vi "VCI Transmit.vi"(6 "Len":u32, 7 "pSend":T1, 8 "error in (no error)":errorcluster, 9 "CANIndex":u32, 10 "DevIndex":u32, 11 "DevType":u32) -> (0 "error out":errorcluster, 3 "function return":u32)   [LabVIEW 2012, in "ControlCAN.lvlib"]
doc: "unsigned int WINAPI VCI_Transmit(unsigned int DevType,unsigned int DevIndex,unsigned int CANIndex,PVCI_CAN_OBJ pSend,unsigned int Len);"
uses:
  ControlCAN.lvlib
  Ginkgo_Driver.dll
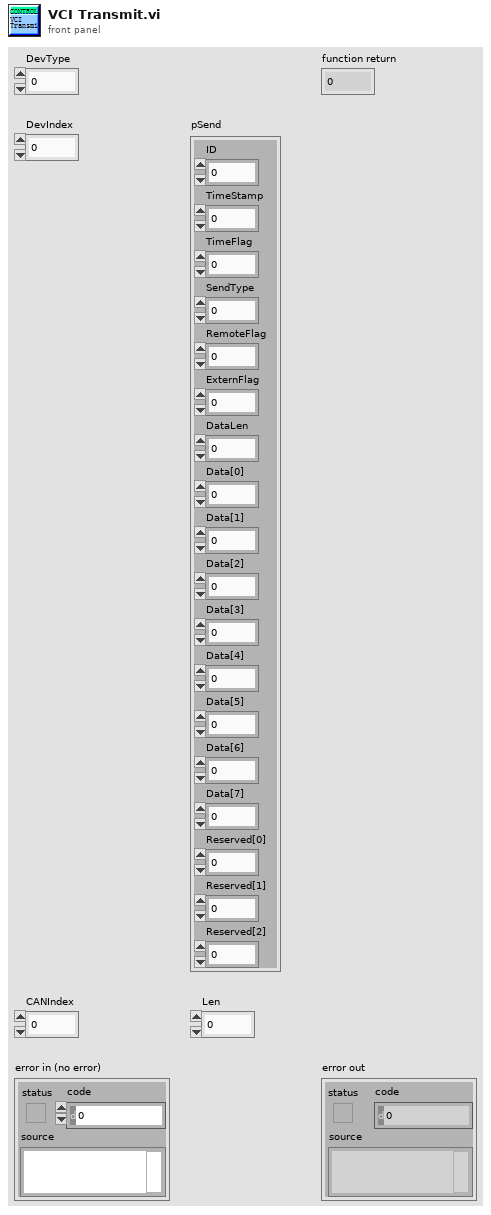
[diagram p1: front panel]
types:
  T1 = cluster{"ID":u32, "TimeStamp":u32, "TimeFlag":u8, "SendType":u8, "RemoteFlag":u8, "ExternFlag":u8, "DataLen":u8, "Data[0]":u8, "Data[1]":u8, "Data[2]":u8, "Data[3]":u8, "Data[4]":u8, "Data[5]":u8, "Data[6]":u8, "Data[7]":u8, "Reserved[0]":u8, "Reserved[1]":u8, "Reserved[2]":u8}
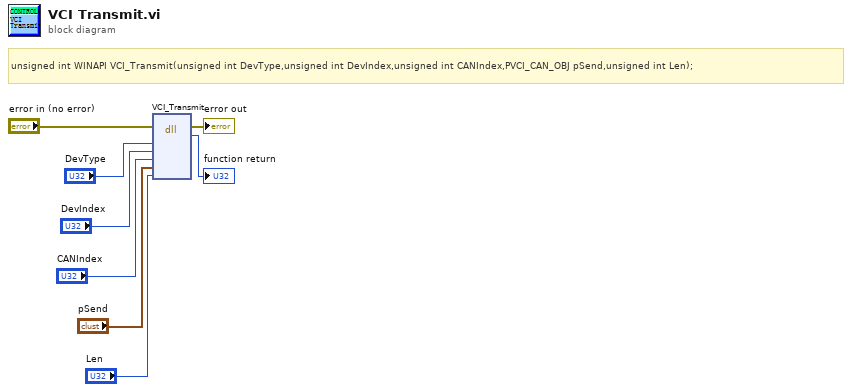
[diagram p0: block diagram]
diagram:
  # "unsigned int WINAPI VCI_Transmit(unsigned int DevType,unsigned int DevIndex,unsigned int CANIndex,PVCI_CAN_OBJ pSend,unsigned int Len);"
  n1 = dll-call lib="E:/Project/vt_ginkgo/truck/Ginkgo Driver/vs2010/Ginkgo_USB-I2C_API_v2.0.3.0/lib/labview_32bit/ControlCAN/Ginkgo_Driver.*" fn="VCI_Transmit"(error in="error in (no error)", "DevType"="DevType", "DevIndex"="DevIndex", "CANIndex"="CANIndex", "pSend"="pSend", "Len"="Len") -> (error out=→"error out":errorcluster, →"function return":u32)  [unwired: 7 in, 1 out]
